vi "updateCaptions.vi"(8 "error in (no error)":errorcluster, 11 "uiControlsMgr in":refnum<class "uiControlsMgr.lvclass">) -> (0 "error out":errorcluster, 3 "uiControlsMgr out":refnum<class "uiControlsMgr.lvclass">)   [LabVIEW 2019, in "uiControlsMgr.lvclass"]
uses:
  uiControlsMgr.lvclass
  uiControlsMgr.lvclass/uiControlsMgr.ctl
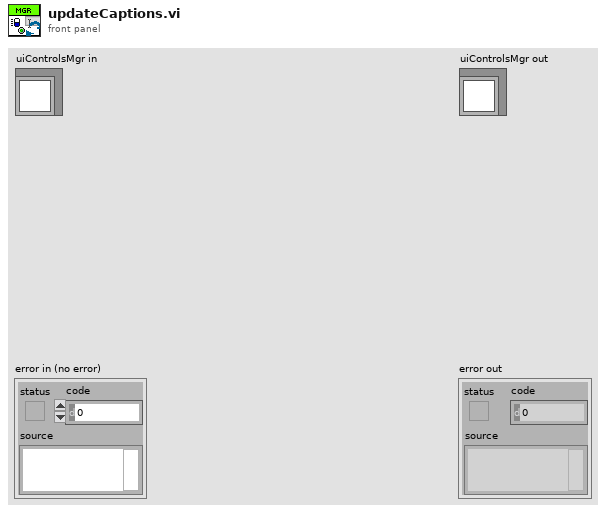
[diagram p1: front panel]
types:
  T1 = map{string, cluster{"Caption":string, "Ctl Refnum":refnum<vi>}}
  T2 = cluster{"Caption":string, "Ctl Refnum":refnum<vi>}
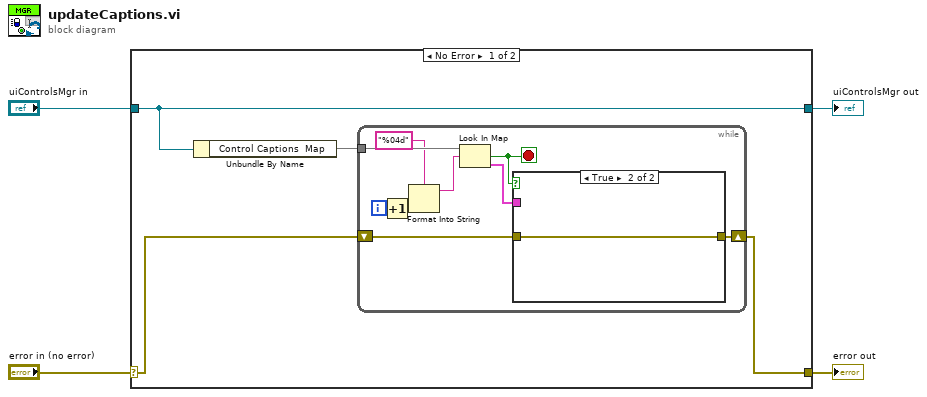
[diagram p0: block diagram]
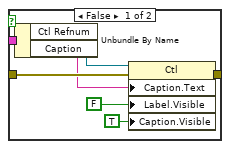
[diagram p2: hidden frame]
diagram:
  n1 = case shown="No Error" "error in (no error)" {
    selector: "error in (no error)" -> [w8 w27]
    tunnel: [w6 w27] -> w3
    tunnel: [w7 w26] -> w1
    tunnel: "uiControlsMgr in" -> [w7 w26]
    frame No Error {
      n2 = Unbundle By Name(w7) -> ("Control Captions  Map"=w5:T1)
      n3 = while {
        shift-right: [w15] -> w6
        shift-left: w8 -> [w17]
        tunnel: w5 -> [w16]
        i -> [w11]
        stop <- w9 stop-if-true
        n4 = Increment(x=w11) -> (x+1=w10:i32)
        n5 = Format Into String(format string="%04d", w10) -> (resulting string=w12:string)  [unwired: 2 in, 1 out]
        n6 = Look In Map(map=w16, key=w12) -> (key not found?=w9:bool, value=w14:T2)  [unwired: 1 in]
        n7 = case shown="True" w9 {
          tunnel: w17 -> [w24 w25]
          tunnel: [w23 w25] -> w15
          tunnel: w14 -> [w22 _]
          frame False {
            n8 = Unbundle By Name(w22) -> ("Ctl Refnum"=w18:refnum<vi>, "Caption"=w19:string)
            n9 = property class="Ctl"(reference=w18, error in=w24, "Caption.Text"=w19, "Label.Visible"=FALSE, "Caption.Visible"=TRUE) -> (error out=w23:errorcluster)  [unwired: 1 out]
          }
          frame True {
          }
        }
      }
    }
    frame Error {
    }
  }
  "error out" <- w3
  "uiControlsMgr out" <- w1
